vi "Get_INI_File_keyValues.vi"(0 "key":string="Calibrator", 2 "name or relative path":string="ModisEdgeMFG.ini", 3 "error in (no error)":errorcluster) -> (7 "value":string, 9 "Key-Value Array":cluster{"value":string}[][](array[cluster])=[[{"value"="Calibrator"}, {"value"="COM12"}], [{"value"="DMM"}, {"value"="COM2"}], [{"value"="Device_names"}, {"value"="Dev1"}], [{"value"="StationID"}, {"value"="TSModisEdge"}], [{"value"="Fixture_SN"}, {"value"="ModisEdgeScopeFixture1"}], [{"value"="AlwaysPrint"}, {"value"="False"}], [{"value"="TestReportPath"}, {"value"="C:\\Snap-On\\ModisEdge_Scope\\"}], [{"value"="ManufactDate"}, {"value"="03-17-2015"}], [{"value"="ManufactLocation"}, {"value"="NeoTech"}], [{"value"="PcbAssemblyNum"}, {"value"="EAP0226L50A"}], [{"value"="PcbRevision"}, {"value"="B"}], [{"value"="LastCalLocation"}, {"value"="NeoTech"}], [{"value"="Delay(s)"}, {"value"="3"}]], 10 "error out":errorcluster)   [LabVIEW 2015]
uses:
  <vilib>/Utility/config.llb/Read Key (String).vi
  <vilib>/Utility/config.llb/NI_LVConfig.lvlib
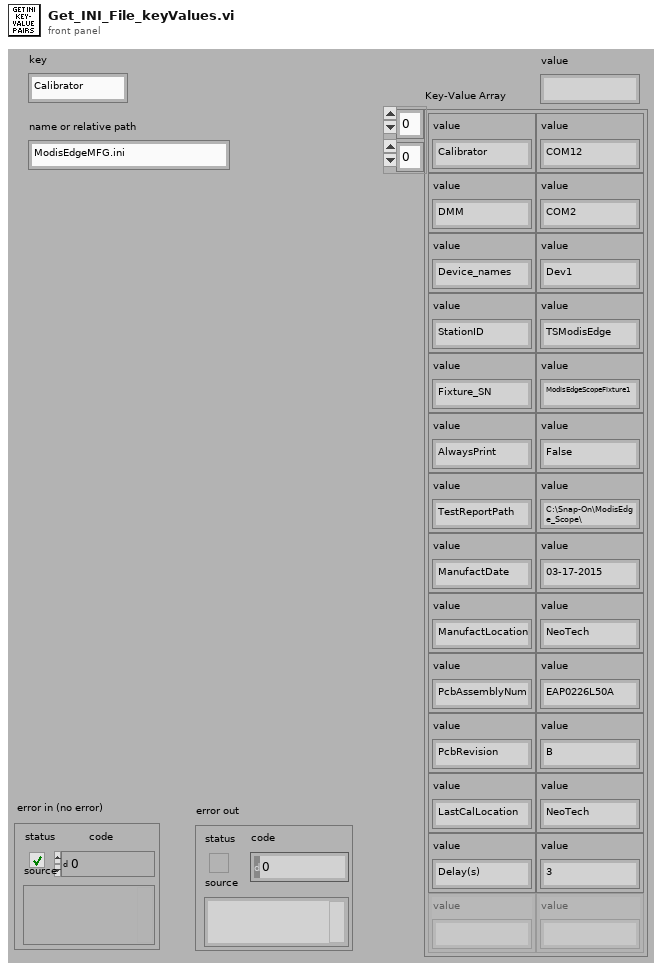
[diagram p1: front panel]
types:
  T1 = typedef "NI_LVConfig.lvlib/Config Data RefNum.ctl" = refnum<k1>
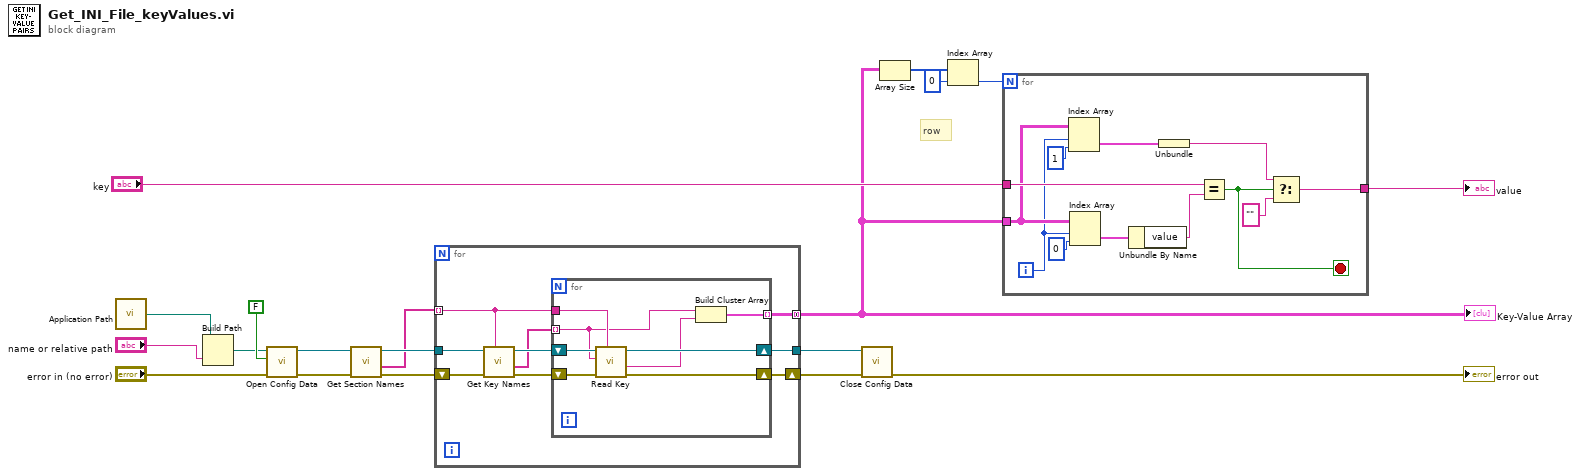
[diagram p0: block diagram]
diagram:
  # "row"
  n1 = call "Application Path.vi"() -> ("path"=w15:path)  [unwired: 5 in]
  n2 = Build Path(base path=w15, name or relative path="name or relative path") -> (appended path=w16:path)
  n3 = call <vilib>:"Open Config Data.vi"("error in (no error)"="error in (no error)", "create file if necessary (T)"=FALSE, "configuration file path"=w16) -> ("error out"=w18:errorcluster, "refnum"=w11:T1)  [unwired: 6 in, 1 out]
  n4 = call <vilib>:"Get Section Names.vi"("error in (no error)"=w18, "refnum"=w11) -> ("error out"=w13:errorcluster, "section names"=w9:string[], "refnum out"=w10:T1)  [unwired: 7 in]
  n5 = for {
    tunnel: w10 -> [w26]
    shift-right: [w25] -> w12
    shift-left: w13 -> [w28]
    tunnel: w9 -> [w22] mode=indexing
    tunnel: [w23] -> w8
    tunnel: [w20] -> w5 mode=concatenating
    n6 = call <vilib>:"Get Key Names.vi"("section"=w22, "error in (no error)"=w28, "refnum"=w26) -> ("error out"=w27:errorcluster, "key names"=w21:string[], "refnum out"=w24:T1)  [unwired: 5 in, 1 out]
    n7 = for {
      shift-right: [w35] -> w25
      shift-left: w27 -> [w36]
      shift-right: [w33] -> w23
      shift-left: w24 -> [w34]
      tunnel: w22 -> [w32]
      tunnel: w21 -> [w31] mode=indexing
      tunnel: [w29] -> w20 mode=indexing
      n8 = call-poly <vilib>:"Read Key.vi"("section"=w32, "error in (no error)"=w36, "key"=w31, "refnum"=w34) -> ("error out"=w35:errorcluster, "value"=w30:string, "refnum out"=w33:T1)  [unwired: 4 in, 1 out]
      n9 = Build Cluster Array(w31, w30) -> (w29:cluster{"value":string}[])
    }
  }
  "Key-Value Array" <- w5
  n10 = call <vilib>:"Close Config Data.vi"("error in (no error)"=w12, "refnum"=w8) -> ("error out"=→"error out":errorcluster)  [unwired: 8 in, 1 out]
  n11 = Array Size(array=w5) -> (size(s)=w4:i32[])
  n12 = Index Array(array=w4, index=0) -> (element=w2:i32)
  n13 = for {
    N: w2 -> [_]
    tunnel: "key" -> [w46]
    tunnel: w5 -> [w44]
    tunnel: [w38] -> w1
    i -> [w43]
    stop <- w37 stop-if-true
    n14 = Index Array(array=w44, index (row)=w43, index (col)=1 ("disabled index (col)")) -> (element=w41:cluster{"value":string})
    n15 = Index Array(array=w44, index (row)=w43, index (col)=0 ("disabled index (col)")) -> (element=w47:cluster{"value":string})
    n16 = Unbundle By Name(w47) -> ("value"=w45:string)
    n17 = Unbundle(w41) -> ("value"=w40:string)
    n18 = Equal?(x=w46, y=w45) -> (x = y?=w37:bool)
    n19 = Select(t=w40, s=w37, f="") -> (s? t:f=w38:string)
  }
  "value" <- w1
